vi "SoftFrontPanel.vi"(8 "error in (no error)":errorcluster, 11 "Digitizer Instrument":refnum<class "Digitizer Instrument.lvclass">) -> (0 "error out":errorcluster, 3 "Digitizer Instrument out":refnum<class "Digitizer Instrument.lvclass">)   [LabVIEW 2025, in "Digitizer.lvlib" / "Digitizer Instrument.lvclass"]
doc: "Copyright 2017 National Instruments Corporation\n\nLicensed under the Apache License, Version 2.0 (the \"License\"); you may not use this file except in compliance with the License. You may obtain a copy of the License at http://www.apache.org/licenses/LICENSE-2.0\nUnless required by applicable law or agreed to in writing, software distributed under the License is distributed on an \"AS IS\" BASIS, WITHOUT WARRANTIES OR CONDITIONS OF ANY KIND, either express or implied. See the License for the specific language governing permissions and limitations under the License."
uses:
  Digitizer Instrument.lvclass
  C:/Users/Public/Documents/Sandia National Labs/TSS Plugin/Abstract Engine.lvlibp/Abstract Instrument/Abstract Instrument.lvclass
  Digitizer Instrument.lvclass/Digitizer Instrument.ctl
  <vilib>/Analysis/baseanly.llb/Mean (DBL).vi
  Digitizer configuration/Digitizer configuration.lvclass
  C:/Users/Public/Documents/Sandia National Labs/TSS Plugin/Abstract Engine.lvlibp/Instrument configuration/Instrument configuration.lvclass
  Users/Public/Documents/Sandia National Labs/TSS Plugin/Abstract Engine.lvlibp/Instrument configuration/Read Instrument Setting.vi
  <vilib>/Analysis/NI_AALBase.lvlib
panel:
  out "Channels":T1(array[cluster]) {"Measurement" format="%#_4p"}
  out "Instrument":string caption="Instrument ::"
  # "ch"
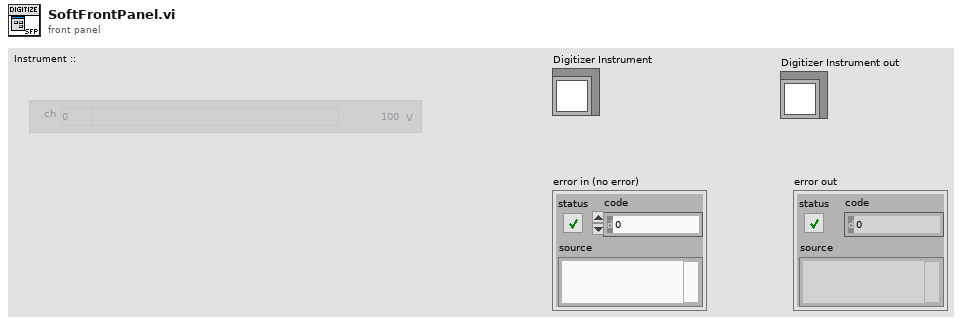
[diagram p1: front panel]
types:
  T1 = cluster{"Channel Alias":string, "Index":i32, "Measurement":dbl}[]
  T2 = enum32{"Invalid", "Default", "Floating", "Floating/Auto-Hide", "Modal"}
  T3 = typedef "Abstract Engine.lvlibp/Instrument configuration.lvclass/Default Instrument.ctl" = cluster{"Type":string, "Address":string, "SW Alias":string, "Description":string, "Enabled":bool}
  T4 = cluster{"Channel Alias":string, "Index":i32, "Measurement":dbl}
  T5 = typedef "Abstract Engine.lvlibp/Abstract Instrument.lvclass/Channel.ctl" = cluster{"Alias":string, "DataType":enum16{"Anaolg Input", "Waveform"}, "Unit":enum16{"---", "V", "A", "Ohm", "Hz", "uF", "degC", "deg"}, "Upper limit":dbl, "Lower limit":dbl, "Measurement":variant}
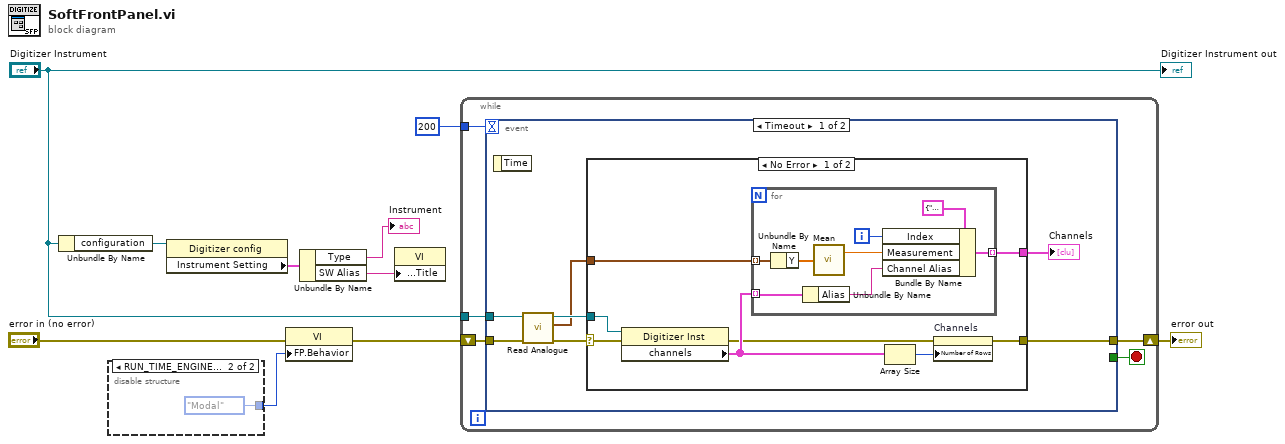
[diagram p0: block diagram]
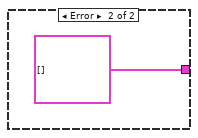
[diagram p2: hidden frame]
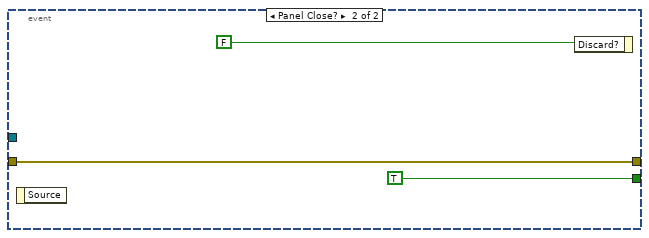
[diagram p3: hidden frame]
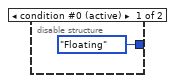
[diagram p4: hidden frame]
diagram:
  n1 = Unbundle By Name("Digitizer Instrument") -> ("configuration"=w7:refnum<class "Digitizer configuration.lvclass">)
  n2 = disable-structure shown="RUN_TIME_ENGINE==True" {
    disable-tunnel: [T2."Floating" ("Front Panel Window:Behavior") T2."Modal" ("Front Panel Window:Behavior")] -> w9
    frame condition #0 (active) {
    }
    frame condition #1 {
    }
  }
  n3 = property class="Digitizer config"(reference=w7) -> ("Instrument Setting"=w6:T3)  [unwired: 1 in, 2 out]
  n4 = property class="VI"(error in="error in (no error)", "FP.Behavior"=w9) -> (error out=w8:errorcluster)  [unwired: 1 in, 1 out]
  n5 = Unbundle By Name(w6) -> ("Type"=→"Instrument":string, "SW Alias"=w5:string)
  n6 = property class="VI"("Front Panel.Title"=w5) -> ()  [unwired: 2 in, 2 out]
  n7 = while {
    shift-right: [w15] -> w1
    shift-left: w8 -> [w16]
    tunnel: 200 -> [w13]
    tunnel: "Digitizer Instrument" -> [w14]
    stop <- w17 stop-if-true
    n8 = event shown="[0] Timeout" {
      selector: _ -> [_ _]
      dyn-events: _ -> [_ _]
      timeout: w13 -> [_ _]
      tunnel: [_ TRUE] -> w17
      tunnel: [w23 w42] -> w15
      tunnel: w16 -> [w21 w42]
      tunnel: w14 -> [w22 _]
      event Timeout {
        n9 = event-data() -> ()  [unwired: 1 in, 1 out]
        n10 = call-dynamic "Read Analogue.vi"("error in (no error)"=w21, "Digitizer Instrument"=w22) -> ("error out"=w20:errorcluster, "Waveforms"=w18:waveform(dbl)[], "Digitizer Instrument out"=w19:refnum<class "Digitizer Instrument.lvclass">)  [unwired: 7 in]
        n11 = case shown="No Error" w20 {
          selector: w20 -> [w26 _]
          tunnel: [w32 T1 []] -> w24
          tunnel: [w28 _] -> w23
          tunnel: w19 -> [w27 _]
          tunnel: w18 -> [w25 _]
          frame No Error {
            n12 = property class="Digitizer Inst"(reference=w27, error in=w26) -> (error out=w29:errorcluster, "channels"=w30:T5[])  [unwired: 1 out]
            n13 = for {
              tunnel: [w40] -> w32 mode=indexing
              tunnel: w25 -> [w39] mode=indexing
              tunnel: w30 -> [w36] mode=indexing
              i -> [w33]
              n14 = Unbundle By Name(w39) -> ("Y"=w38:dbl[])
              n15 = Unbundle By Name(w36) -> ("Alias"=w35:string)
              n16 = call-poly <vilib>:"Mean.vi"("X"=w38) -> ("mean"=w37:dbl)  [unwired: 1 out]
              n17 = Bundle By Name(cluster=T4 {"Channel Alias"="", "Index"=0, "Measurement"=nan} ("Channel"), "Index"=w33, "Measurement"=w37, "Channel Alias"=w35) -> (w40:T4)
            }
            n18 = Array Size(array=w30) -> (size(s)=w31:i32)
            n19 = property on="Channels" class="Arr (strict)"(error in=w29, "Number of Rows"=w31) -> (error out=w28:errorcluster)  [unwired: 1 in, 1 out]
          }
          frame Error {
          }
        }
        "Channels" <- w24
      }
      event Panel Close? {
        n20 = event-data() -> ()  [unwired: 1 in, 1 out]
        n21 = event-data("Discard?"=FALSE) -> ()  [unwired: 1 in, 1 out]
      }
    }
  }
  "error out" <- w1
  "Digitizer Instrument out" <- "Digitizer Instrument"
